vi "testFailIndicator.vi"() -> ()   [LabVIEW 2011, in "No Object Control TestCase.lvclass"]
uses:
  No Object Control TestCase.lvclass
panel:
  out "Fail":bool=TRUE
  out "error out":errorcluster
  in  "error in (no error)":errorcluster
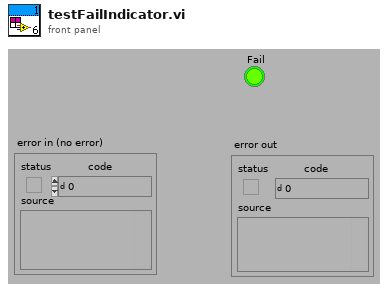
[diagram p1: front panel]
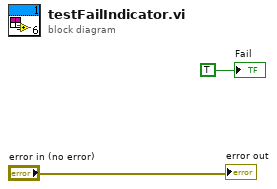
[diagram p0: block diagram]
diagram:
  "error out" <- "error in (no error)"
  "Fail" <- TRUE ("Fail")
